vi "Example 2.vi"() -> ()   [LabVIEW 2016]
uses:
  <vilib>/express/express arith-compare/Formula/XNode/ExpressFormulaBlockNode.xnode
panel:
  out "V":dbl
  out "SA":dbl
  out "A":dbl
  out "C":dbl
  in  "H":dbl
  in  "r inches":dbl
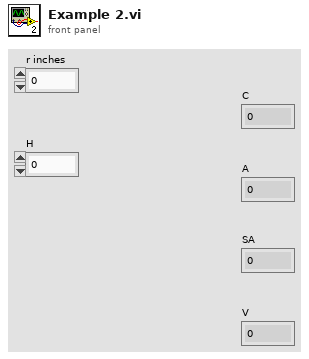
[diagram p1: front panel]
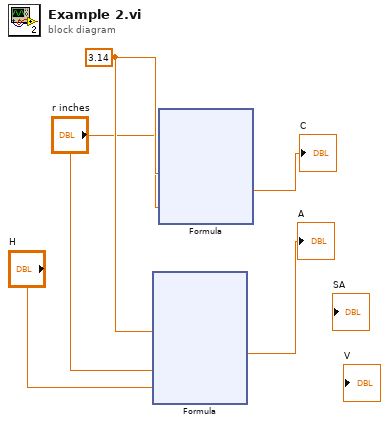
[diagram p0: block diagram]
diagram:
  w4 = 3.14
  n1 = xnode "Formula"("pi"=w4, "r"="r inches", "h"="H") -> ("Result"=→"A":dbl)  [unwired: 1 in, 1 out]
  n2 = xnode "Formula"("pi"=w4, "r"="r inches") -> ("Result"=→"C":dbl)  [unwired: 1 in, 1 out]
